vi "Draw_SGP.vi"(0 "y":dbl[](array[numeric]), 4 "PicAjust":T2={"TranslationVector"=[], "scale"=1.0, "Pitch（x) "=0.0, "Yaw（y)"=0.0, "Roll（z) "=0.0} {"Roll（z)" scale=-90.0..90.0; "Yaw（y)" scale=-90.0..90.0; "Pitch（x)" scale=-90.0..90.0}, 5 "视图":enum16{"俯视图", "轴测图"}(ring), 6 "PathM":dbl[][](array[numeric])=[[50.0, 50.0, 500.0], [500.0, 50.0, 500.0], [500.0, 350.0, 500.0], [50.0, 350.0, 500.0], [50.0, 50.0, 500.0]], 7 "StartPoint":dbl[](array[numeric])=[50.0, 50.0, 500.0], 8 "Image In 2":T1, 9 "Image In 1":T1) -> (1 "x+y":dbl[](array[numeric]), 2 "Image Out 2":T1, 3 "Image Out 1":T1)   [LabVIEW 2014]
doc: "在二维图中显示起点终点以及路径"
uses:
  <vilib>/vision/Image Controls.llb/IMAQ Image.ctl
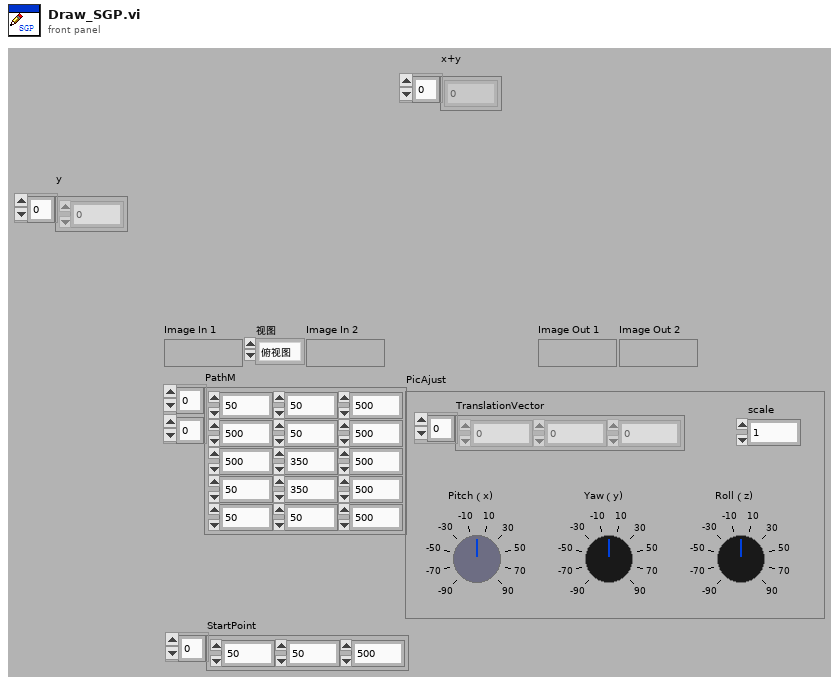
[diagram p1: front panel]
types:
  T1 = typedef "IMAQ Image.ctl" = refnum<image>
  T2 = cluster{"TranslationVector":dbl[], "scale":dbl, "Pitch（x) ":dbl, "Yaw（y)":dbl, "Roll（z) ":dbl}
  T3 = cluster{"StartPoint[0]":dbl, "StartPoint[1]":dbl}
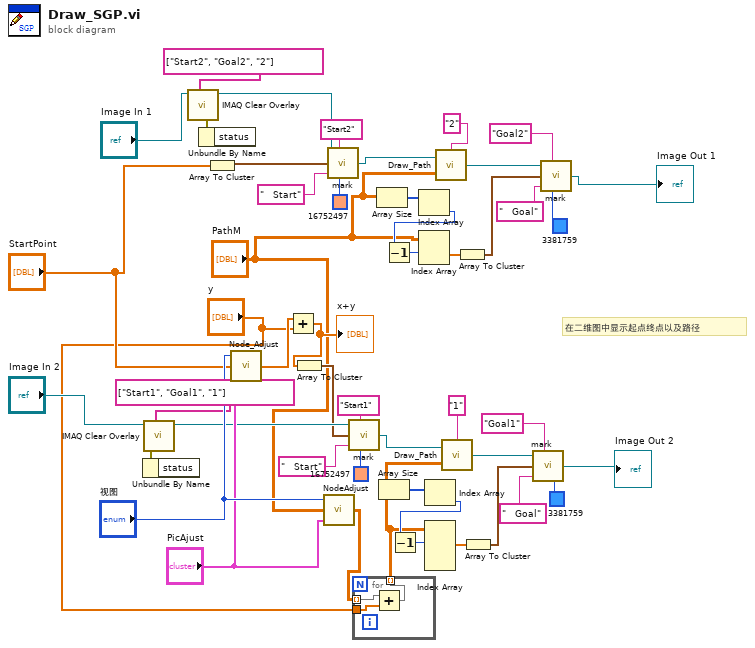
[diagram p0: block diagram]
diagram:
  # "在二维图中显示起点终点以及路径"
  n1 = call "IMAQ Clear Overlay"("Groups"=string[] ["Start1", "Goal1", "1"], "Image"="Image In 2") -> ("error out"=w22:errorcluster, "Image Out"=w15:T1)  [unwired: 8 in]
  n2 = Unbundle By Name(w22) -> ()  [unwired: 1 out]
  n3 = call "IMAQ Clear Overlay"("Groups"=string[] ["Start2", "Goal2", "2"], "Image"="Image In 1") -> ("error out"=w23:errorcluster, "Image Out"=w19:T1)  [unwired: 8 in]
  n4 = Unbundle By Name(w23) -> ()  [unwired: 1 out]
  n5 = Array To Cluster(array="StartPoint") -> (cluster=w26:T3)
  n6 = call "Node_Adjust.vi"("PicAjust"="PicAjust", "Node"="StartPoint", "视图"="视图") -> ("NewNode"=w6:dbl[])
  n7 = Add(x=w6, y="y") -> (x+y=w5:dbl[])
  "x+y" <- w5
  n8 = Array To Cluster(array=w5) -> (cluster=w7:cluster{"[0]":dbl, "[1]":dbl})
  n9 = call "NodeAdjust.vi"("PicAjust"="PicAjust", "NodeM"="PathM", "视图"="视图") -> ("NewNodeM"=w3:dbl[][])
  n10 = call "mark.vi"("Image In"=w19, "Group"="Start2", "Point"=w26, "String"="   Start", "Text Color (black)"=u32 16752497) -> ("Image Out"=w18:T1)
  n11 = call "mark.vi"("Image In"=w15, "Group"="Start1", "Point"=w7, "String"="   Start", "Text Color (black)"=u32 16752497) -> ("Image Out"=w14:T1)
  n12 = for {
    tunnel: w3 -> [w52] mode=indexing
    tunnel: "y" -> [w51]
    tunnel: [w50] -> w2 mode=indexing
    n13 = Add(x=w52, y=w51) -> (x+y=w50:dbl[])
  }
  n14 = Array Size(array="PathM") -> (size(s)=w49:i32[])
  n15 = Array Size(array=w2) -> (size(s)=w42:i32[])
  n16 = Index Array(array=w49) -> (element=w46:i32)  [unwired: 1 in]
  n17 = Decrement(x=w46) -> (x-1=w47:i32)
  n18 = Index Array(array="PathM", index (row)=w47) -> (element=w48:dbl[])  [unwired: 1 in]
  n19 = Index Array(array=w42) -> (element=w45:i32)  [unwired: 1 in]
  n20 = Decrement(x=w45) -> (x-1=w44:i32)
  n21 = Index Array(array=w2, index (row) #1=w44) -> (element #1=w43:dbl[])  [unwired: 3 in, 1 out]
  n22 = call "Draw_Path.vi"("Group"="2", "PathM"="PathM", "Image Out 2"=w18) -> ("Image Out"=w33:T1)
  n23 = call "Draw_Path.vi"("Group"="1", "PathM"=w2, "Image Out 2"=w14) -> ("Image Out"=w31:T1)
  n24 = Array To Cluster(array=w48) -> (cluster=w32:cluster{"PathM[0]":dbl, "PathM[1]":dbl})
  n25 = Array To Cluster(array=w43) -> (cluster=w30:cluster{"[0]":dbl, "[1]":dbl})
  n26 = call "mark.vi"("Image In"=w31, "Group"="Goal1", "Point"=w30, "String"="   Goal", "Text Color (black)"=u32 3381759) -> ("Image Out"=→"Image Out 2":T1)
  n27 = call "mark.vi"("Image In"=w33, "Group"="Goal2", "Point"=w32, "String"="   Goal", "Text Color (black)"=u32 3381759) -> ("Image Out"=→"Image Out 1":T1)
